vi "Camera.vi"(7 "Machine Vision":T1=enum."Tray Fiducials", 8 "error in (no error)":errorcluster, 10 "Stop":bool, 11 "Camera in":refnum<class "Camera.lvclass">) -> (0 "error out":errorcluster, 1 "Camera":dbl[](array[numeric]), 2 "Image":T2(plugin-control), 3 "Camera out":refnum<class "Camera.lvclass">)   [LabVIEW 2016, in "Camera.lvclass"]
uses:
  Camera.lvclass
  Machine Vision.ctl
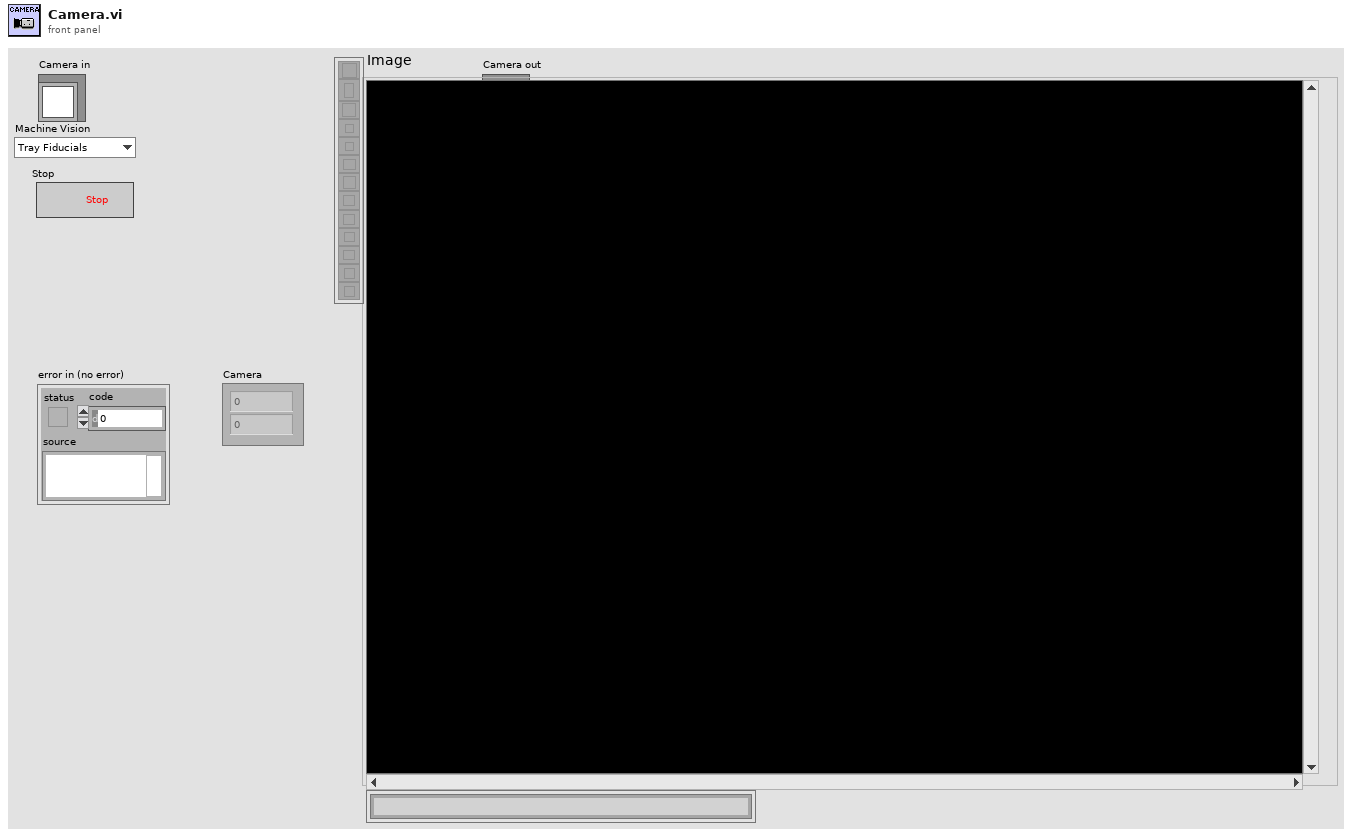
[diagram p1: front panel]
types:
  T1 = typedef "Camera.lvclass/Machine Vision.ctl" = enum16{"None", "Circle", "Tray Fiducials", "Tray Fiducials, top right", "HPK Silicon square", "HPK Silicon", "8inch PCB Pad", "Hexaboard", "Corner (TL, BR)", "Corner (BL, TR)"}
  T2 = typedef "IMAQ Image.ctl" = refnum<image>
  T3 = typedef "IMAQ GM Match Report.ctl" = cluster{"Position":cluster{"x":sgl, "y":sgl}, "Angle":sgl, "Scale":sgl, "Score":sgl, "Bounding Box":cluster{"x":sgl, "y":sgl}[], "Contrast Reversed":bool, "Occlusion %":sgl, "Template Target Curve Score":sgl, "Target Template Curve Score":sgl, "Correlation Score":sgl}
  T4 = cluster{"Center (Pixels)":cluster{"X":sgl, "Y":sgl}, "Radius (Pixels)":dbl, "Center (Real-World)":cluster{"X":sgl, "Y":sgl}, "Radius (Real-World)":dbl, "Roundness (Real-World)":dbl, "Average Strength":dbl, "Average SNR (dB)":dbl}
  T5 = cluster{"Position":cluster{"x":sgl, "y":sgl}, "Angle":sgl, "Scale":sgl, "Score":sgl, "Bounding Box":cluster{"x":sgl, "y":sgl}[]}[]
  T6 = cluster{"Position":cluster{"x":sgl, "y":sgl}, "Angle":sgl, "Scale":sgl, "Score":sgl, "Bounding Box":cluster{"x":sgl, "y":sgl}[]}
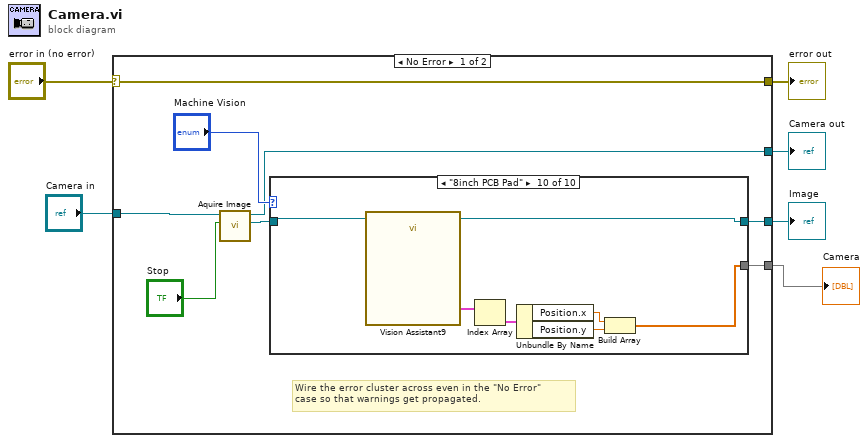
[diagram p0: block diagram]
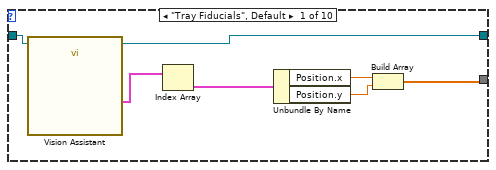
[diagram p2: hidden frame]
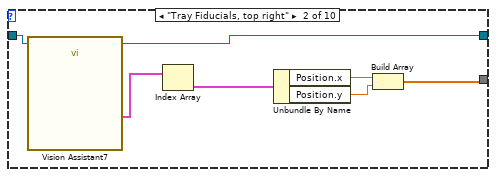
[diagram p3: hidden frame]
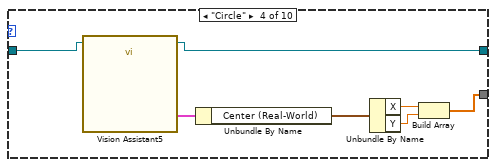
[diagram p5: hidden frame]
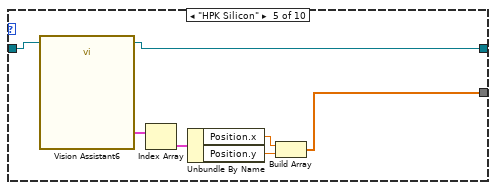
[diagram p6: hidden frame]
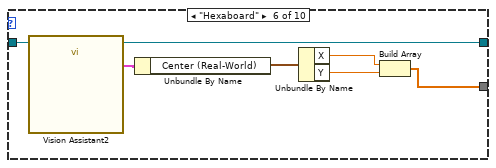
[diagram p7: hidden frame]
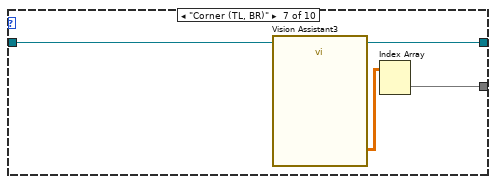
[diagram p8: hidden frame]
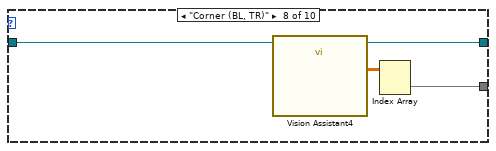
[diagram p9: hidden frame]
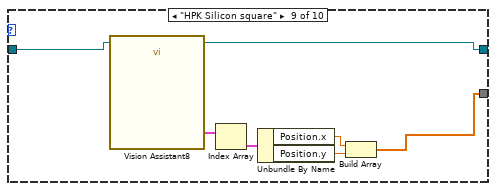
[diagram p10: hidden frame]
diagram:
  n1 = case shown="No Error" "error in (no error)" {
    selector: "error in (no error)" -> [w14 w74]
    tunnel: [w14 w74] -> w5
    tunnel: [w10 w73] -> w4
    tunnel: "Camera in" -> [w11 w73]
    tunnel: [w9 _] -> w2
    tunnel: [w8 _] -> w1
    frame No Error {
      # "Wire the error cluster across even in the \"No Error\"\ncase so that warnings get propagated."
      n2 = call-dynamic "Aquire Image.vi"("Stop"="Stop", "Camera in"=w11) -> ("Image Out"=w7:T2, "Camera out"=w10:refnum<class "Camera.lvclass">)  [unwired: 7 in, 1 out]
      n3 = case shown="\"8inch PCB Pad\"" "Machine Vision" {
        tunnel: [w15 w22 _ w33 w38 w44 w52 w55 w59 w66] -> w9
        tunnel: [w20 w27 w29 w32 w39 w45 w54 w58 w60 w67] -> w8
        tunnel: w7 -> [w21 w28 w29 w31 w37 w46 w53 w57 w61 w68]
        frame "Tray Fiducials", Default {
          n4 = call "Vision Assistant"("Image In"=w21) -> ("Image Out"=w20:T2, "Calibrated Matches (Geometric Matching 1)"=w16:T3[])  [unwired: 23 in, 2 out]
          n5 = Index Array(array=w16) -> (element=w19:T3)  [unwired: 1 in]
          n6 = Unbundle By Name(w19) -> ("Position.x"=w18:sgl, "Position.y"=w17:sgl)
          n7 = Build Array(w18, w17) -> (w15:sgl[])
        }
        frame "Tray Fiducials, top right" {
          n8 = call "Vision Assistant7"("Image In"=w28) -> ("Image Out"=w27:T2, "Calibrated Matches (Geometric Matching 1)"=w23:T3[])  [unwired: 23 in, 2 out]
          n9 = Index Array(array=w23) -> (element=w26:T3)  [unwired: 1 in]
          n10 = Unbundle By Name(w26) -> ("Position.x"=w25:sgl, "Position.y"=w24:sgl)
          n11 = Build Array(w25, w24) -> (w22:sgl[])
        }
        frame "None" {
        }
        frame "Circle" {
          n12 = call "Vision Assistant5"("Image In"=w31) -> ("Image Out"=w32:T2, "Fitted Circle (Find Circular Edge 1)"=w30:T4)  [unwired: 24 in, 1 out]
          n13 = Unbundle By Name(w30) -> ("Center (Real-World)"=w36:cluster{"X":sgl, "Y":sgl})
          n14 = Unbundle By Name(w36) -> ("X"=w35:sgl, "Y"=w34:sgl)
          n15 = Build Array(w35, w34) -> (w33:sgl[])
        }
        frame "HPK Silicon" {
          n16 = call "Vision Assistant6"("Image In"=w37) -> ("Image Out"=w39:T2, "Calibrated Matches (Geometric Matching 1)"=w40:T3[])  [unwired: 23 in, 2 out]
          n17 = Index Array(array=w40) -> (element=w43:T3)  [unwired: 1 in]
          n18 = Unbundle By Name(w43) -> ("Position.x"=w42:sgl, "Position.y"=w41:sgl)
          n19 = Build Array(w42, w41) -> (w38:sgl[])
        }
        frame "Hexaboard" {
          n20 = call "Vision Assistant2"("Image In"=w46) -> ("Image Out"=w45:T2, "Fitted Circle (Find Circular Edge 1)"=w48:T4)  [unwired: 24 in, 1 out]
          n21 = Unbundle By Name(w48) -> ("Center (Real-World)"=w50:cluster{"X":sgl, "Y":sgl})
          n22 = Unbundle By Name(w50) -> ("X"=w49:sgl, "Y"=w47:sgl)
          n23 = Build Array(w49, w47) -> (w44:sgl[])
        }
        frame "Corner (TL, BR)" {
          n24 = call "Vision Assistant3"("Image In"=w53) -> ("Image Out"=w54:T2, "Calibrated Results (Caliper 1)"=w51:sgl[][])  [unwired: 23 in, 2 out]
          n25 = Index Array(array=w51) -> (element=w52:sgl[])  [unwired: 2 in]
        }
        frame "Corner (BL, TR)" {
          n26 = call "Vision Assistant4"("Image In"=w57) -> ("Image Out"=w58:T2, "Calibrated Results (Bottom Left, Top Right)"=w56:sgl[][])  [unwired: 23 in, 2 out]
          n27 = Index Array(array=w56) -> (element=w55:sgl[])  [unwired: 2 in]
        }
        frame "HPK Silicon square" {
          n28 = call "Vision Assistant8"("Image In"=w61) -> ("Image Out"=w60:T2, "Calibrated Matches (Pattern Matching 1)"=w65:T5)  [unwired: 23 in, 2 out]
          n29 = Index Array(array=w65) -> (element=w62:T6)  [unwired: 1 in]
          n30 = Unbundle By Name(w62) -> ("Position.x"=w63:sgl, "Position.y"=w64:sgl)
          n31 = Build Array(w63, w64) -> (w59:sgl[])
        }
        frame "8inch PCB Pad" {
          n32 = call "Vision Assistant9"("Image In"=w68) -> ("Image Out"=w67:T2, "Calibrated Matches (Pattern Matching 1)"=w72:T5)  [unwired: 23 in, 2 out]
          n33 = Index Array(array=w72) -> (element=w69:T6)  [unwired: 1 in]
          n34 = Unbundle By Name(w69) -> ("Position.x"=w70:sgl, "Position.y"=w71:sgl)
          n35 = Build Array(w70, w71) -> (w66:sgl[])
        }
      }
    }
    frame Error {
    }
  }
  "error out" <- w5
  "Camera out" <- w4
  "Camera" <- w2
  "Image" <- w1
